vi "tcp_sva_handler.vi"(0 "button_tcp_connect":bool, 5 "button_tcp_load_cal":bool, 7 "button_get_trace_data":bool) -> (12 "freq_range":cluster{"data out":string, "data out":string}, 13 "data_out":cluster{"data out":string, "data out":string}, 14 "new_data_available":bool, 15 "error out":errorcluster)   [LabVIEW 2025]
uses:
  a4adc4b4-9dcf-4776-a5cb-d51f6fbe3b33.vi
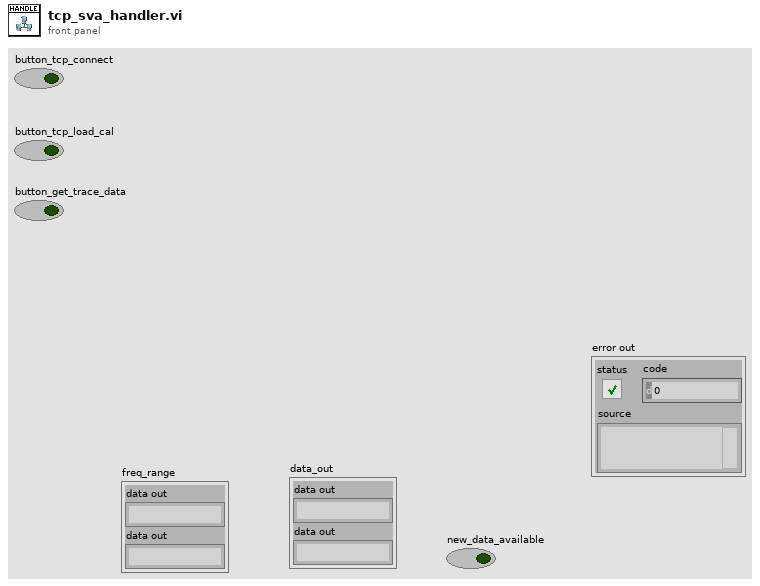
[diagram p1: front panel]
types:
  T1 = cluster{"mode":string, "s11_s21":string, "graph":string, "freq_range":cluster{"start_freq":string, "stop_freq":string}, "points":string}
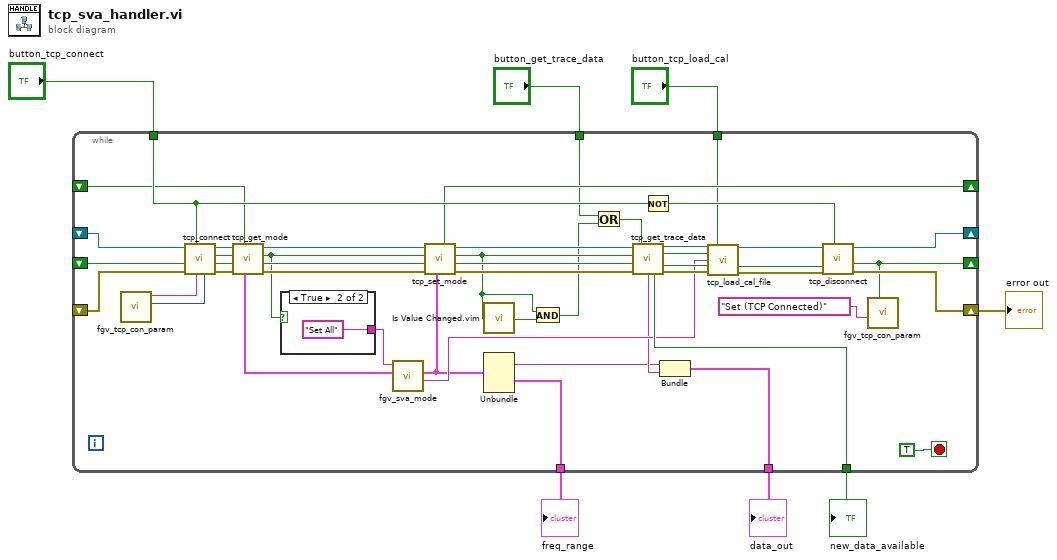
[diagram p0: block diagram]
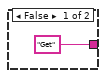
[diagram p2: hidden frame]
diagram:
  n1 = while {
    tunnel: [w14] -> w5
    tunnel: [w12] -> w6
    tunnel: "button_tcp_connect" -> [w39]
    tunnel: [w38] -> w2
    shift-right: [w31] -> _
    shift-left: _ -> [w36]
    shift-right: [w35] -> _
    shift-left: _ -> [w34]
    shift-right: [w32] -> w4
    shift-left: _ -> [w27]
    shift-right: [w26] -> _
    shift-left: _ -> [w25]
    tunnel: "button_tcp_load_cal" -> [w17]
    tunnel: "button_get_trace_data" -> [w8]
    stop <- TRUE stop-if-true
    n2 = call "fgv_tcp_con_param.vi"() -> ("port_get"=w28:u16, "ip_address_get"=w29:string)  [unwired: 8 in, 2 out]
    n3 = call "tcp_connect.vi"("Port"=w28, "IP"=w29, "button_tcp_connect"=w39, "error_in"=w27, "tcp_connected_in"=w36, "connection_id_in"=w25) -> ("error out"=w50:errorcluster, "tcp_connected_out"=w51:bool, "new_connection"=w52:bool, "connection_id_out"=w53:refnum<k5>)  [unwired: 2 in]
    n4 = call "tcp_get_mode.vi"("button_get_mode"=w34, "error in"=w50, "tcp_connected_in"=w51, "new_connection_in"=w52, "connection_id_in"=w53) -> ("error out"=w45:errorcluster, "tcp_connected_out"=w46:bool, "new_data_available"=w33:bool, "connection_id_out"=w47:refnum<k5>, "data_out"=w49:T1)  [unwired: 2 in]
    n5 = case shown="True" w33 {
      tunnel: ["Get" ("mode") "Set All" ("mode")] -> w48
      frame False {
      }
      frame True {
      }
    }
    n6 = call "fgv_sva_mode.vi"("data_in"=w49, "mode"=w48) -> ("cal_file_out"=w16:string, "data_out"=w15:T1)  [unwired: 7 in, 1 out]
    n7 = call "tcp_set_mode.vi"("data_in"=w15, "error in"=w45, "tcp_connected_in"=w46, "new_data_available"=w33, "connection_id_in"=w47) -> ("error out"=w43:errorcluster, "tcp_connected_out"=w42:bool, "sva_ready"=w40:bool, "connection_id_out"=w44:refnum<k5>, "mode_set"=w35:bool)  [unwired: 2 in]
    n8 = call "Is Value Changed.vim"("value"=w40) -> ("changed or first call?"=w41:bool)
    n9 = Unbundle(w15) -> ("s11_s21"=w11:string, "freq_range"=w14:cluster{"start_freq":string, "stop_freq":string})  [unwired: 3 out]
    n10 = And(x=w40, y=w41) -> (x .and. y?=w9:bool)
    n11 = Or(x=w8, y=w9) -> (x .or. y?=w10:bool)
    n12 = call "tcp_get_trace_data.vi"("connection_id_in"=w44, "button_tcp_get_trace"=w10, "sva_ready_in"=w40, "tcp_connected_in"=w42, "error in"=w43) -> ("connection_id_out"=w24:refnum<k5>, "sva_ready_out"=w23:bool, "tcp_connected_out"=w22:bool, "trace_data"=w13:string, "new_data_available"=w38:bool, "error out"=w21:errorcluster)  [unwired: 5 in]
    n13 = Not(x=w39) -> (.not. x?=w54:bool)
    n14 = Bundle("s11_s21"=w11, "trace_data"=w13) -> (w12:cluster{"s11_s21":string, "trace_data":string})  [unwired: 1 in]
    n15 = call "tcp_load_cal_file.vi"("connection_id_in"=w24, "button_tcp_load_cal"=w17, "sva_ready"=w23, "cal_file"=w16, "tcp_connected_in"=w22, "error in"=w21) -> ("connection_id_out"=w20:refnum<k5>, "tcp_connected_out"=w19:bool, "error out"=w18:errorcluster)  [unwired: 7 in]
    n16 = call "tcp_disconnect.vi"("button_tcp_disconnect"=w54, "error in"=w18, "tcp_connected_in"=w19, "connection_id_in"=w20) -> ("error out"=w32:errorcluster, "tcp_connected_out"=w31:bool, "connection_id_out"=w26:refnum<k5>)  [unwired: 5 in]
    n17 = call "fgv_tcp_con_param.vi"("tcp_connected_set"=w31, "mode"="Set (TCP Connected)") -> ()  [unwired: 6 in, 4 out]
  }
  "new_data_available" <- w2
  "error out" <- w4
  "data_out" <- w6
  "freq_range" <- w5
